vi "AC Source manual control GUI.vi"(10 "AC sync source":T1={"AC Source type"=enum."Tektronix AFG3000 series", "VISA"="", "Ref. clock (Hz)"=10000000.0, "status ref"=refnum, "Fluke 57XX wideband output"=FALSE, "Fluke 57XX ignore errors"=FALSE, "Synchronization by AC signal"=FALSE} caption="Synchronization of AC Source\n(Amplitude of this source is set automatically)" {"Ref. clock (Hz)" format="%#_7p"}, 11 "AC Source":T1={"AC Source type"=enum."Tektronix AFG3000 series", "VISA"="", "Ref. clock (Hz)"=10000000.0, "status ref"=refnum, "Fluke 57XX wideband output"=FALSE, "Fluke 57XX ignore errors"=FALSE, "Synchronization by AC signal"=FALSE} {"Ref. clock (Hz)" format="%#_7p"}) -> ()   [LabVIEW 2020]
doc: "GUI to manally controll the AC source."
uses:
  Type definitions/AC Source.ctl
  Type definitions/AC Source type.ctl
  <vilib>/Utility/error.llb/Error Cluster From Error Code.vi
  <vilib>/ErrorRing/Error Ring.xnode
  external libraries/varilib/varilib.lvlib
panel:
  out "error out":errorcluster
  in  "General Settings:Timeout Value":u32=2000
  in  "Signal amplitude (V)":dbl=0.707
  in  "Signal frequency  (Hz)":dbl=1000.0
  in  "stop":bool
  in  "start":bool
  out "gui_elements":refnum<vi>[](array[refnum])
  out "Status":string
  in  "initialize":bool
  in  "quit":bool
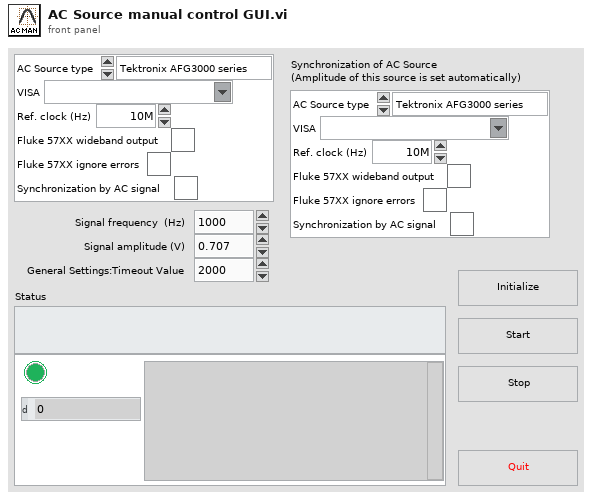
[diagram p1: front panel]
types:
  T1 = typedef "AC Source.ctl" = cluster{"AC Source type":T2, "VISA":refnum<visa-resource-name>, "Ref. clock (Hz)":dbl, "status ref":refnum<vi>, "Fluke 57XX wideband output":bool, "Fluke 57XX ignore errors":bool, "Synchronization by AC signal":bool}
  T2 = typedef "AC Source type.ctl" = enum16{"Fluke 5XXX calibrator", "Tektronix AFG3000 series", "dummy", "Agilent 331xxA to 332xxA", "Agilent 335xxA to 336xxA"}
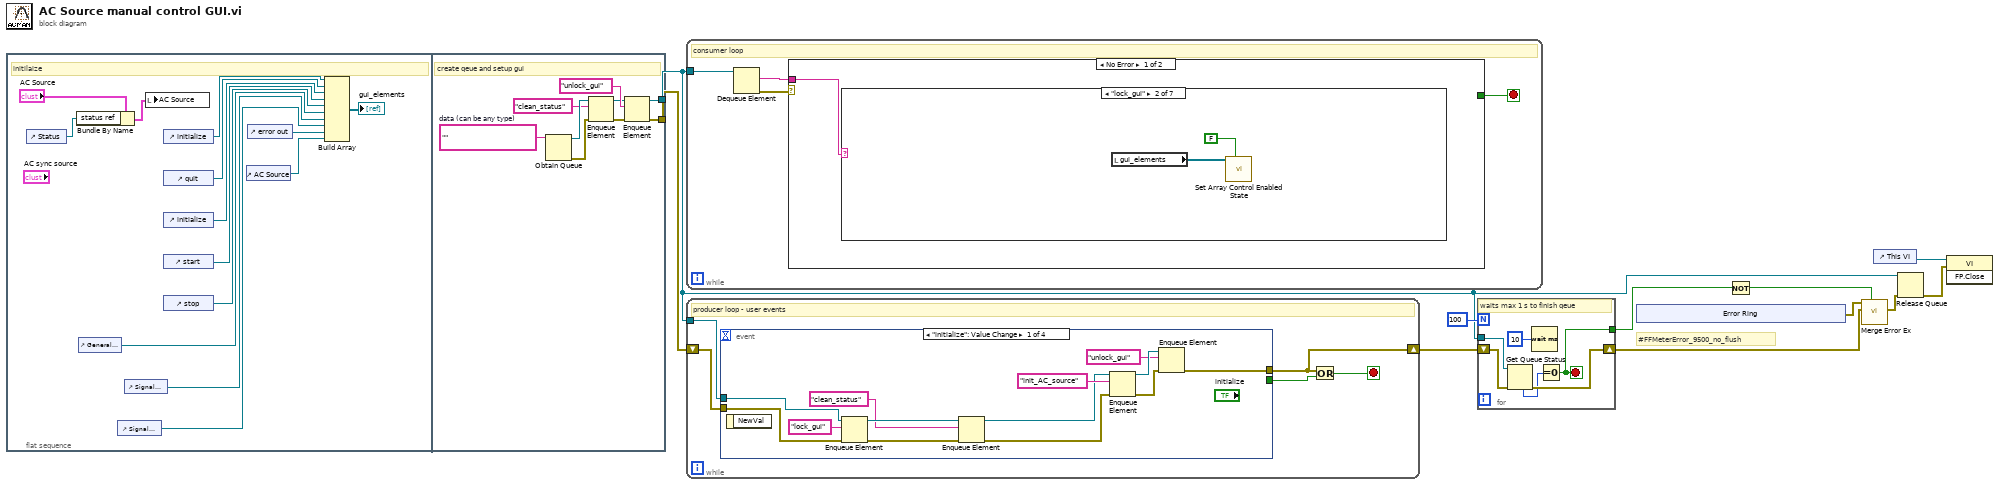
[diagram p0: block diagram]
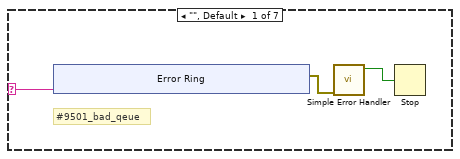
[diagram p2: hidden frame]
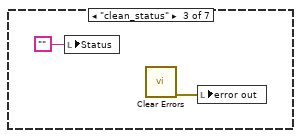
[diagram p3: hidden frame]
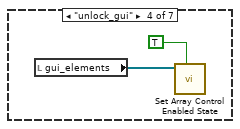
[diagram p4: hidden frame]
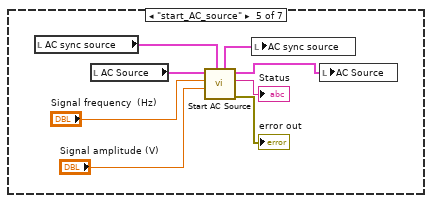
[diagram p5: hidden frame]
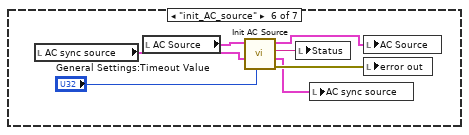
[diagram p6: hidden frame]
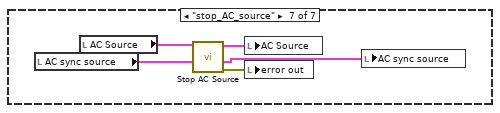
[diagram p7: hidden frame]
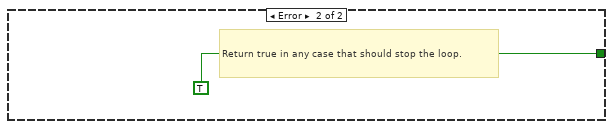
[diagram p8: hidden frame]
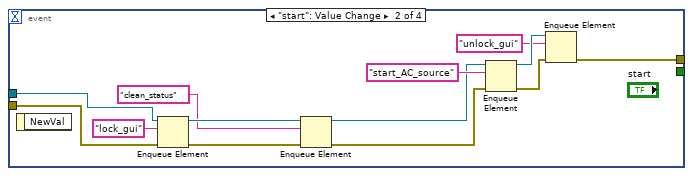
[diagram p9: hidden frame]
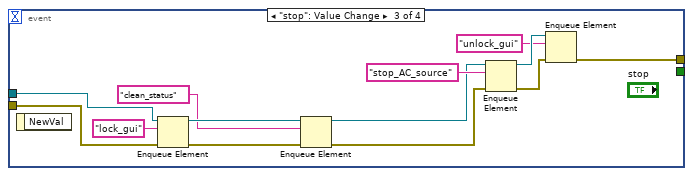
[diagram p10: hidden frame]
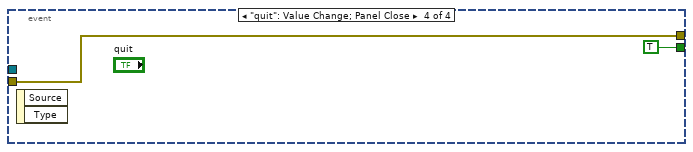
[diagram p11: hidden frame]
diagram:
  # "#FFMeterError_9500_no_flush"
  n1 = flat-sequence {
    tunnel: [w30] -> w4
    tunnel: [w28] -> w3
    frame #0 {
      # "initilaize"
      n2 = control-ref of="Status"() -> (w13:refnum<vi>)
      n3 = Bundle By Name(cluster="AC Source", "status ref"=w13) -> (w12:T1)
      n4 = control-ref of="General Settings:Timeout Value"() -> (w19:refnum<vi>)
      n5 = control-ref of="Signal frequency  (Hz)"() -> (w17:refnum<vi>)
      n6 = control-ref of="Signal amplitude (V)"() -> (w18:refnum<vi>)
      n7 = local write "AC Source"(w12) -> ()
      n8 = control-ref of="initialize"() -> (w25:refnum<vi>)
      n9 = control-ref of="quit"() -> (w24:refnum<vi>)
      n10 = control-ref of="initialize"() -> (w20:refnum<vi>)
      n11 = control-ref of="start"() -> (w21:refnum<vi>)
      n12 = control-ref of="stop"() -> (w22:refnum<vi>)
      n13 = control-ref of="AC Source"() -> (w15:refnum<vi>)
      n14 = control-ref of="error out"() -> (w16:refnum<vi>)
      n15 = Build Array(w25, w24, w20, w21, w22, w19, w18, w17, w16, w15) -> (→"gui_elements":refnum<vi>[])
    }
    frame #1 {
      w29 = ""  # data (can be any type)
      # "create qeue and setup gui"
      n16 = Obtain Queue(element data type=w29) -> (queue out=w33:refnum<queue>, error out=w34:errorcluster)  [unwired: 4 in, 1 out]
      n17 = Enqueue Element(queue=w33, element="clean_status", error in (no error)=w34) -> (queue out=w26:refnum<queue>, error out=w27:errorcluster)  [unwired: 1 in, 1 out]
      n18 = Enqueue Element(queue=w26, element="unlock_gui", error in (no error)=w27) -> (queue out=w30:refnum<queue>, error out=w28:errorcluster)  [unwired: 1 in, 1 out]
    }
  }
  n19 = while {
    tunnel: w4 -> [w38]
    stop <- w35 stop-if-true
    # "consumer loop"
    n20 = Dequeue Element(queue=w38) -> (element=w36:string, error out=w37:errorcluster)  [unwired: 2 in, 2 out]
    n21 = case shown="No Error" w37 {
      tunnel: w36 -> [w39 _]
      tunnel: [_ TRUE] -> w35
      frame No Error {
        n22 = case shown="\"lock_gui\"" w39 {
          selector: w39 -> [w40 _ _ _ _ _ _]
          frame "", Default {
            # "#9501_bad_qeue"
            n23 = xnode "Error Ring"("parameter 0"=w40) -> ("error out"=w42:errorcluster)
            n24 = call <vilib>:"Simple Error Handler.vi"("error in (no error)"=w42) -> ("error?"=w41:bool)  [unwired: 4 in, 4 out]
            n25 = Stop(stop? (T)=w41) -> ()
          }
          frame "lock_gui" {
            n26 = local read "gui_elements"() -> (w51:refnum<vi>[])
            n27 = call "Set Array Control Enabled State.vi"("enabled (T)"=FALSE, "reference array in"=w51) -> ()  [unwired: 8 in, 2 out]
          }
          frame "clean_status" {
            n28 = local write "Status"("") -> ()
            n29 = call <vilib>:"Clear Errors.vi"() -> ("error out"=w52:errorcluster)  [unwired: 6 in, 1 out]
            n30 = local write "error out"(w52) -> ()
          }
          frame "unlock_gui" {
            n31 = local read "gui_elements"() -> (w55:refnum<vi>[])
            n32 = call "Set Array Control Enabled State.vi"("enabled (T)"=TRUE, "reference array in"=w55) -> ()  [unwired: 8 in, 2 out]
          }
          frame "start_AC_source" {
            n33 = local read "AC sync source"() -> (w57:T1)
            n34 = local read "AC Source"() -> (w63:T1)
            n35 = call "Start AC Source.vi"("AC sync source"=w57, "Signal amplitude (V)"="Signal amplitude (V)", "Signal frequency  (Hz)"="Signal frequency  (Hz)", "AC source"=w63) -> ("error out"=→"error out":errorcluster, "status"=→"Status":string, "AC source out"=w62:T1, "AC sync source out"=w56:T1)  [unwired: 4 in]
            n36 = local write "AC sync source"(w56) -> ()
            n37 = local write "AC Source"(w62) -> ()
          }
          frame "init_AC_source" {
            n38 = local read "AC sync source"() -> (w65:T1)
            n39 = local read "AC Source"() -> (w70:T1)
            n40 = call "Init AC Source.vi"("General Settings:Timeout Value"="General Settings:Timeout Value", "AC sync source"=w65, "AC source"=w70) -> ("error out"=w66:errorcluster, "AC sync source out"=w64:T1, "Init status"=w68:string, "AC source out"=w69:T1)  [unwired: 5 in]
            n41 = local write "Status"(w68) -> ()
            n42 = local write "AC sync source"(w64) -> ()
            n43 = local write "AC Source"(w69) -> ()
            n44 = local write "error out"(w66) -> ()
          }
          frame "stop_AC_source" {
            n45 = local read "AC sync source"() -> (w71:T1)
            n46 = local read "AC Source"() -> (w74:T1)
            n47 = call "Stop AC Source.vi"("AC sync source"=w71, "AC source"=w74) -> ("error out"=w75:errorcluster, "AC sync source out"=w72:T1, "AC source out"=w73:T1)  [unwired: 7 in]
            n48 = local write "AC Source"(w73) -> ()
            n49 = local write "error out"(w75) -> ()
            n50 = local write "AC sync source"(w72) -> ()
          }
        }
      }
      frame Error {
        # "Return true in any case that should stop the loop."
      }
    }
  }
  n51 = while {
    shift-right: [w77] -> w7
    shift-left: w3 -> [w80]
    tunnel: w4 -> [w81]
    stop <- w78 stop-if-true
    # "producer loop - user events"
    n52 = event shown="[0] \"initialize\": Value Change" {
      selector: _ -> [_ _ _ _]
      dyn-events: _ -> [_ _ _ _]
      timeout: _ -> [_ _ _ _]
      tunnel: w81 -> [w88 w101 w114 _]
      tunnel: w80 -> [w89 w102 w115 w122]
      tunnel: [w92 w105 w118 w122] -> w77
      tunnel: [_ _ _ TRUE ("cancel")] -> w79
      event "initialize": Value Change {
        n53 = event-data() -> ()  [unwired: 1 in, 1 out]
        n54 = Enqueue Element(queue=w88, element="lock_gui", error in (no error)=w89) -> (queue out=w85:refnum<queue>, error out=w86:errorcluster)  [unwired: 1 in, 1 out]
        n55 = Enqueue Element(queue=w85, element="clean_status", error in (no error)=w86) -> (queue out=w83:refnum<queue>, error out=w82:errorcluster)  [unwired: 1 in, 1 out]
        n56 = Enqueue Element(queue=w83, element="init_AC_source", error in (no error)=w82) -> (queue out=w91:refnum<queue>, error out=w93:errorcluster)  [unwired: 1 in, 1 out]
        n57 = Enqueue Element(queue=w91, element="unlock_gui", error in (no error)=w93) -> (error out=w92:errorcluster)  [unwired: 1 in, 2 out]
      }
      event "start": Value Change {
        n58 = event-data() -> ()  [unwired: 1 in, 1 out]
        n59 = Enqueue Element(queue=w101, element="lock_gui", error in (no error)=w102) -> (queue out=w98:refnum<queue>, error out=w99:errorcluster)  [unwired: 1 in, 1 out]
        n60 = Enqueue Element(queue=w98, element="clean_status", error in (no error)=w99) -> (queue out=w96:refnum<queue>, error out=w95:errorcluster)  [unwired: 1 in, 1 out]
        n61 = Enqueue Element(queue=w96, element="start_AC_source", error in (no error)=w95) -> (queue out=w104:refnum<queue>, error out=w106:errorcluster)  [unwired: 1 in, 1 out]
        n62 = Enqueue Element(queue=w104, element="unlock_gui", error in (no error)=w106) -> (error out=w105:errorcluster)  [unwired: 1 in, 2 out]
      }
      event "stop": Value Change {
        n63 = event-data() -> ()  [unwired: 1 in, 1 out]
        n64 = Enqueue Element(queue=w114, element="lock_gui", error in (no error)=w115) -> (queue out=w111:refnum<queue>, error out=w112:errorcluster)  [unwired: 1 in, 1 out]
        n65 = Enqueue Element(queue=w111, element="clean_status", error in (no error)=w112) -> (queue out=w109:refnum<queue>, error out=w108:errorcluster)  [unwired: 1 in, 1 out]
        n66 = Enqueue Element(queue=w109, element="stop_AC_source", error in (no error)=w108) -> (queue out=w117:refnum<queue>, error out=w119:errorcluster)  [unwired: 1 in, 1 out]
        n67 = Enqueue Element(queue=w117, element="unlock_gui", error in (no error)=w119) -> (error out=w118:errorcluster)  [unwired: 1 in, 2 out]
      }
      event "quit": Value Change; Panel Close {
        n68 = event-data() -> ()  [unwired: 1 in, 2 out]
      }
    }
    n69 = Or(x=w77, y=w79) -> (x .or. y?=w78:bool)
  }
  n70 = for {
    N: 100 -> [_]
    tunnel: w4 -> [w128]
    shift-right: [w126] -> w8
    shift-left: w7 -> [w127]
    tunnel: [w123] -> w5
    stop <- w123 stop-if-true
    # "waits max 1 s to finish qeue"
    n71 = Get Queue Status(queue=w128, error in (no error)=w127) -> (error out=w126:errorcluster, # elements in queue=w124:i32)  [unwired: 1 in, 6 out]
    n72 = Wait (ms)(milliseconds to wait=u32 10) -> ()  [unwired: 1 out]
    n73 = Equal To 0?(x=w124) -> (x = 0?=w123:bool)
  }
  n74 = xnode "Error Ring"() -> ("error out"=w9:errorcluster)
  n75 = Not(x=w5) -> (.not. x?=w10:bool)
  n76 = call "Merge Error Ex.vi"("Is error? (False)"=w10, "main error in (no error)"=w8, "second error in"=w9) -> ("error out"=w6:errorcluster)  [unwired: 8 in]
  n77 = control-ref of="This VI"() -> (w2:refnum<vi>)
  n78 = Release Queue(queue=w4, error in (no error)=w6) -> (error out=w1:errorcluster)  [unwired: 1 in, 2 out]
  n79 = invoke class="VI" method="FP.Close"(reference=w2, error in=w1) -> ()  [unwired: 1 in, 3 out]
